vi "cm2nm_read_session_data_file_backup.vi"(2 "TopLevelDataFilePath":path, 3 "Session_data_base":path) -> (0 "error out":errorcluster, 1 "Sample Set":T6)   [LabVIEW 2010]
uses:
  cm2nm_sample_set.ctl
  cm2nm_coordinate_information_v2.ctl
  Instrument_type_enum_v2.ctl
  cm2nm_sample_set_old_1.ctl
  Instrument_type_enum.ctl
  <vilib>/Utility/xml.llb/Read From XML File(string).vi
panel:
  out "Sample Set 4":T1
  out "Sample Set 3":T4
  in  "Sample Set 2":T5
  out "String":string
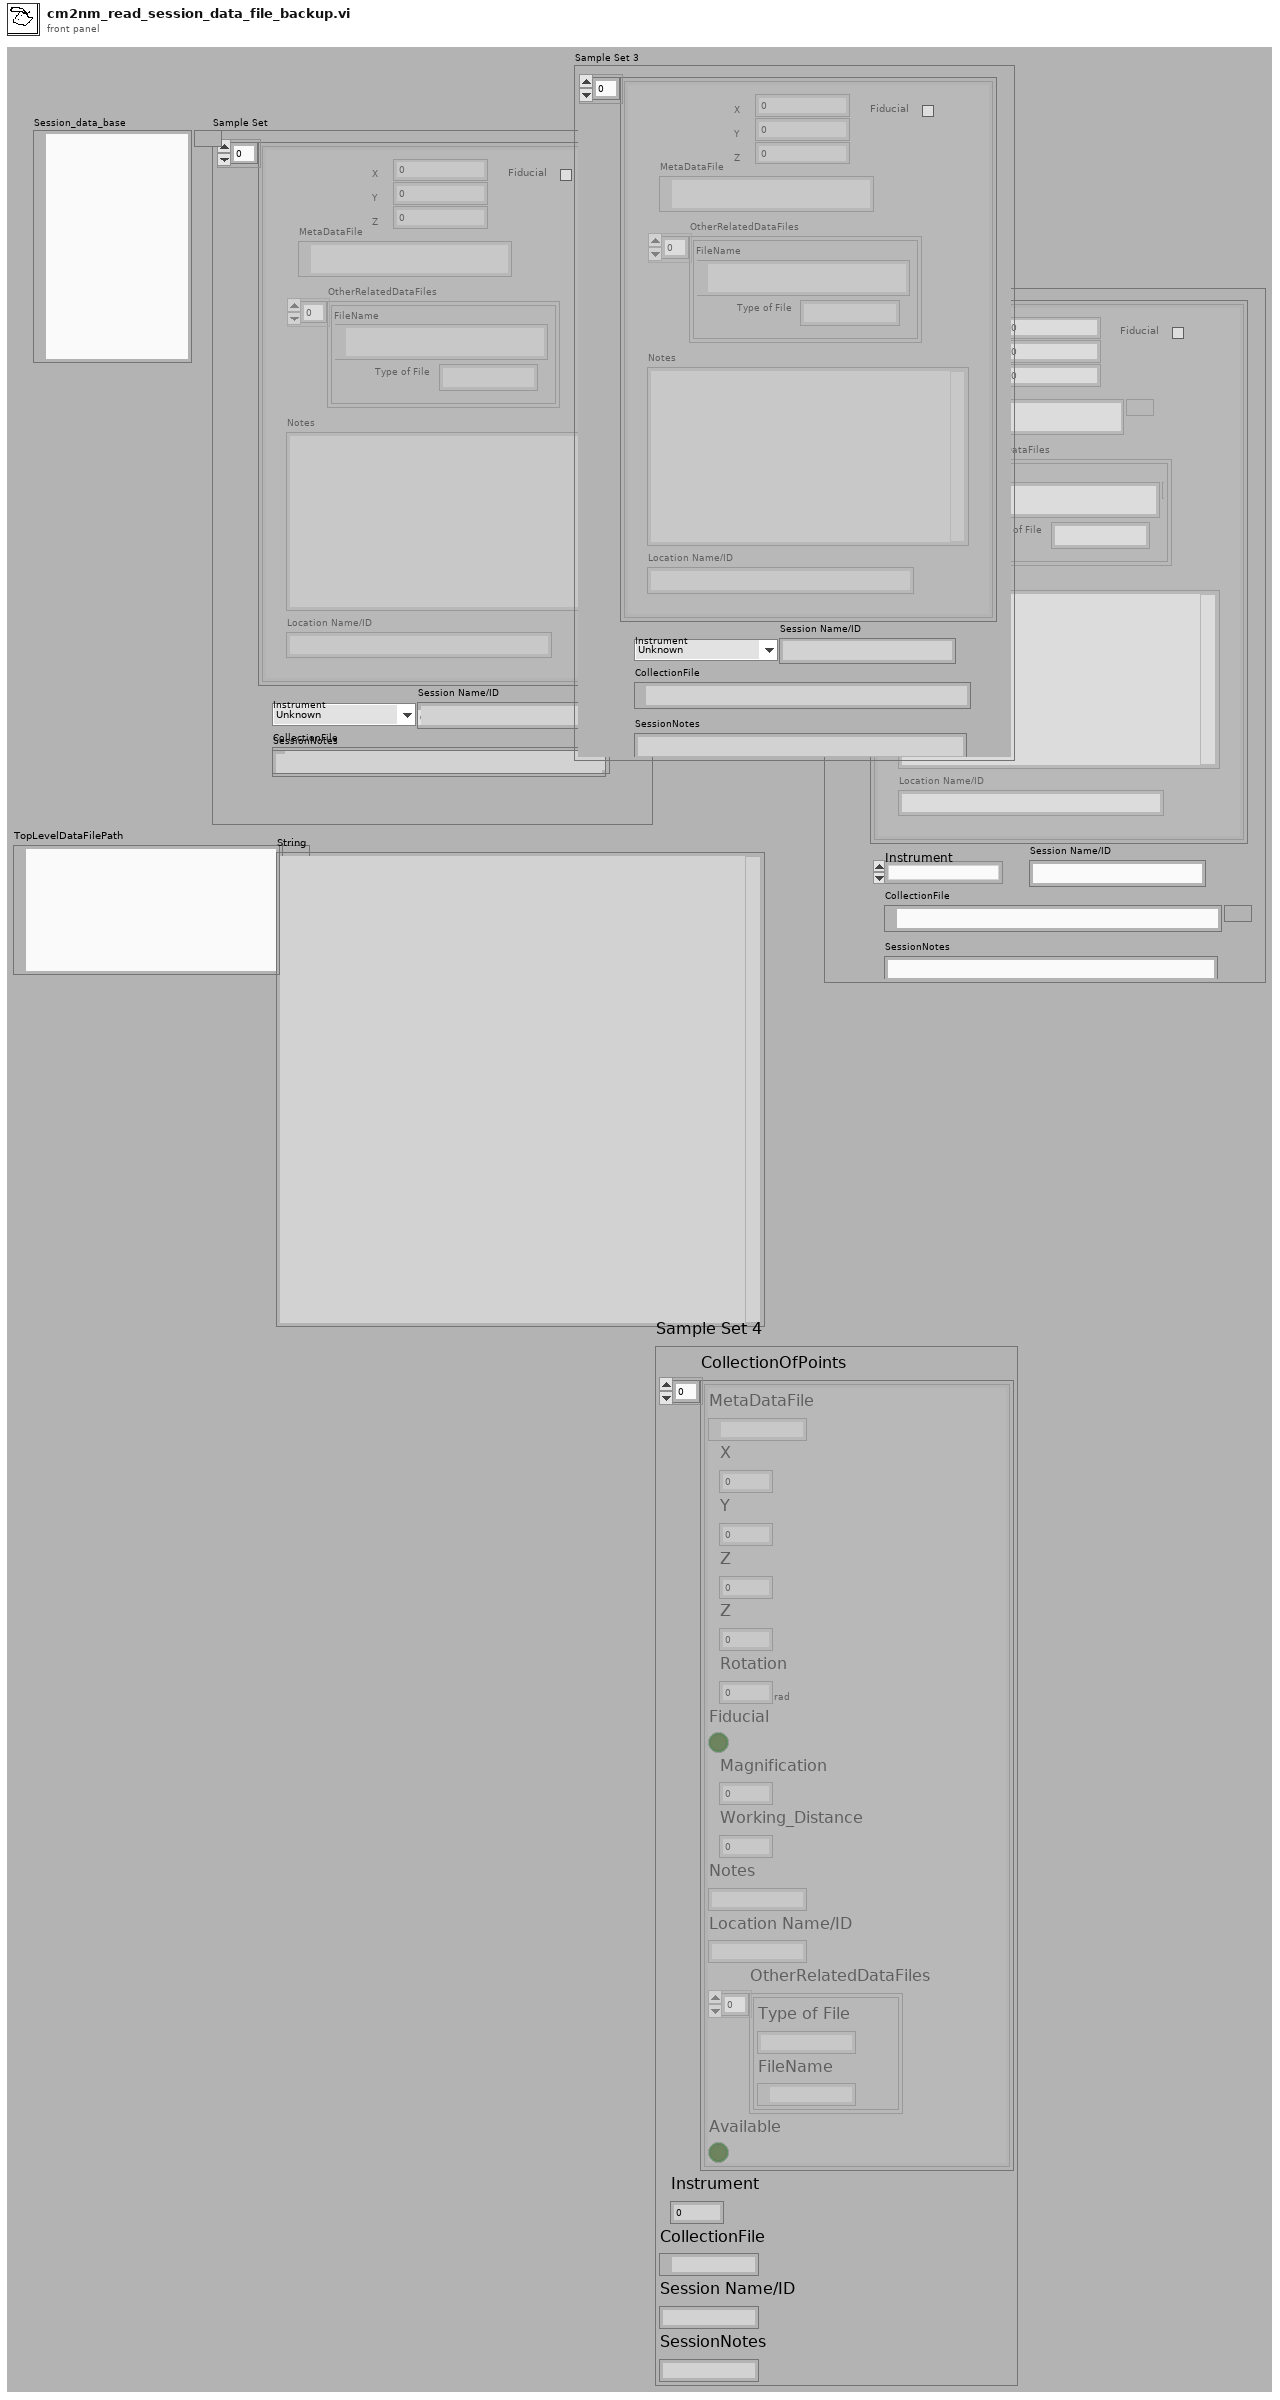
[diagram p1: front panel]
types:
  T1 = cluster{"CollectionOfPoints":cluster{"MetaDataFile":path, "X":dbl, "Y":dbl, "Z":dbl, "Z":dbl, "Rotation":dbl[unit], "Fiducial":bool, "Magnification":dbl, "Working_Distance":dbl, "Notes":string, "Location Name/ID":string, "OtherRelatedDataFiles":cluster{"Type of File":string, "FileName":path}[], "Available":bool}[], "Instrument":u16, "CollectionFile":path, "Session Name/ID":string, "SessionNotes":string}
  T2 = typedef "cm2nm_coordinate_information_v2.ctl" = cluster{"MetaDataFile":path, "X":dbl, "Y":dbl, "Z":dbl, "Group":i32, "Rotation":dbl[unit], "Fiducial":bool, "Magnification":dbl, "Working_Distance":dbl, "Notes":string, "Location Name/ID":string, "OtherRelatedDataFiles":cluster{"Type of File":string, "FileName":path}[], "Available":bool}
  T3 = typedef "Instrument_type_enum.ctl" = enum16{"Unknown", "Phillips FEI SEM IRC", "JEOL 7000F EML_MFC", "MXRD MFC", "JEOL_EPMA"}
  T4 = cluster{"CollectionOfPoints":T2[], "Instrument":T3, "CollectionFile":path, "Session Name/ID":string, "SessionNotes":string}
  T5 = typedef "cm2nm_sample_set_old_1.ctl" = cluster{"CollectionOfPoints":T2[], "Instrument":enum16{""}, "CollectionFile":path, "Session Name/ID":string, "SessionNotes":string}
  T6 = typedef "cm2nm_sample_set.ctl" = cluster{"CollectionOfPoints":T2[], "Instrument":T7, "CollectionFile":path, "Session Name/ID":string, "SessionNotes":string}
  T7 = typedef "Instrument_type_enum_v2.ctl" = enum16{"Unknown", "Philips FEI SEM IRC", "JEOL 7000F EML_MFC", "MXRD MFC", "JEOL_EPMA"}
  T8 = cluster{"CollectionOfPoints":cluster{"MetaDataFile":path, "X":dbl, "Y":dbl, "Group":i32, "Z":dbl, "Rotation":dbl[unit], "Fiducial":bool, "Magnification":dbl, "Working_Distance":dbl, "Notes":string, "Location Name/ID":string, "OtherRelatedDataFiles":cluster{"Type of File":string, "FileName":path}[], "Available":bool}[], "Instrument":T7, "CollectionFile":path, "Session Name/ID":string, "SessionNotes":string}
  T9 = cluster{"CollectionOfPoints":cluster{"MetaDataFile":path, "X":dbl, "Y":dbl, "Z":dbl, "Group":i32, "Rotation":dbl[unit], "Fiducial":bool, "Magnification":dbl, "Working_Distance":dbl, "Notes":string, "Location Name/ID":string, "OtherRelatedDataFiles":cluster{"Type of File":string, "FileName":path}[], "Available":bool}[], "Instrument":T3, "CollectionFile":path, "Session Name/ID":string, "SessionNotes":string}
  T10 = cluster{"MetaDataFile":path, "X":dbl, "Y":dbl, "Z":dbl, "Group":i32, "Rotation":dbl[unit], "Fiducial":bool, "Magnification":dbl, "Working_Distance":dbl, "Notes":string, "Location Name/ID":string, "OtherRelatedDataFiles":cluster{"Type of File":string, "FileName":path}[], "Available":bool}[]
  T11 = cluster{"MetaDataFile":path, "X":dbl, "Y":dbl, "Group":i32, "Z":dbl, "Rotation":dbl[unit], "Fiducial":bool, "Magnification":dbl, "Working_Distance":dbl, "Notes":string, "Location Name/ID":string, "OtherRelatedDataFiles":cluster{"Type of File":string, "FileName":path}[], "Available":bool}[]
  T12 = cluster{"CollectionOfPoints":cluster{"MetaDataFile":path, "X":dbl, "Y":dbl, "Group":i32, "Z":dbl, "Rotation":dbl[unit], "Fiducial":bool, "Magnification":dbl, "Working_Distance":dbl, "Notes":string, "Location Name/ID":string, "OtherRelatedDataFiles":cluster{"Type of File":string, "FileName":path}[], "Available":bool}[], "Instrument":u16, "CollectionFile":path, "Session Name/ID":string, "SessionNotes":string}
  T13 = cluster{"MetaDataFile":path, "X":dbl, "Y":dbl, "Z":dbl, "Z":dbl, "Rotation":dbl[unit], "Fiducial":bool, "Magnification":dbl, "Working_Distance":dbl, "Notes":string, "Location Name/ID":string, "OtherRelatedDataFiles":cluster{"Type of File":string, "FileName":path}[], "Available":bool}[]
  T14 = cluster{"MetaDataFile":path, "X":dbl, "Y":dbl, "Z":dbl, "Z":dbl, "Rotation":dbl[unit], "Fiducial":bool, "Magnification":dbl, "Working_Distance":dbl, "Notes":string, "Location Name/ID":string, "OtherRelatedDataFiles":cluster{"Type of File":string, "FileName":path}[], "Available":bool}
  T15 = cluster{"CollectionOfPoints":cluster{"MetaDataFile":path, "X":dbl, "Y":dbl, "Z":dbl, "Z":dbl, "Rotation":dbl[unit], "Fiducial":bool, "Magnification":dbl, "Working_Distance":dbl, "Notes":string, "Location Name/ID":string, "OtherRelatedDataFiles":cluster{"Type of File":string, "FileName":path}[], "Available":bool}[], "Instrument":T7, "CollectionFile":path, "Session Name/ID":string, "SessionNotes":string}
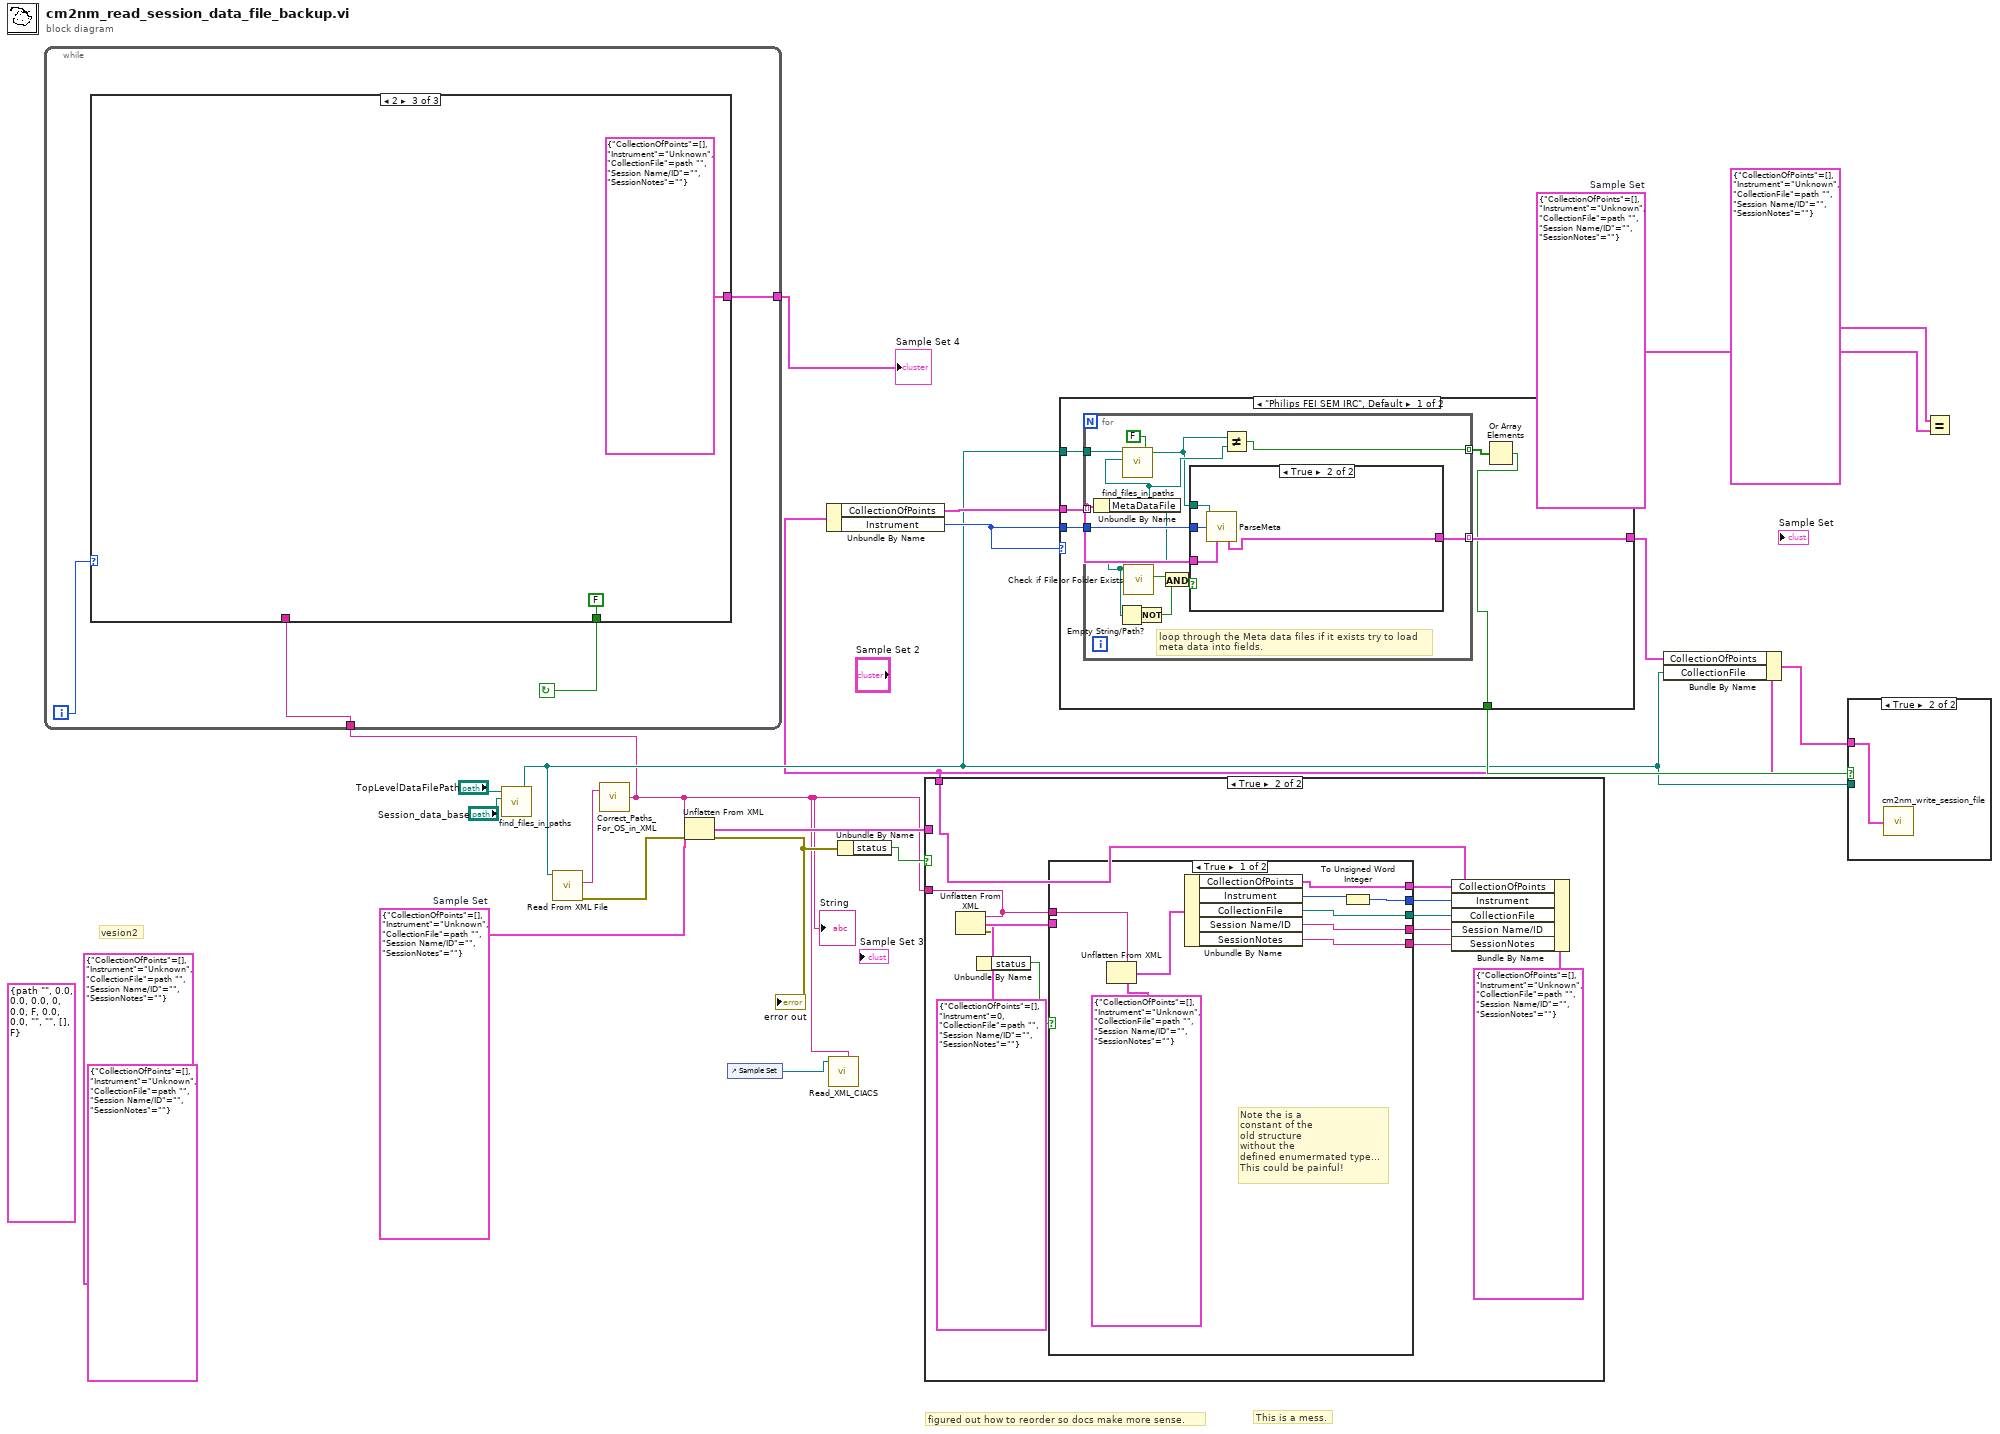
[diagram p0: block diagram]
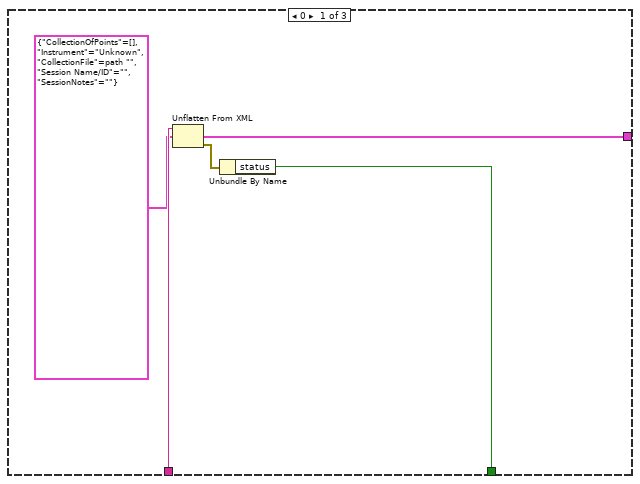
[diagram p2: hidden frame]
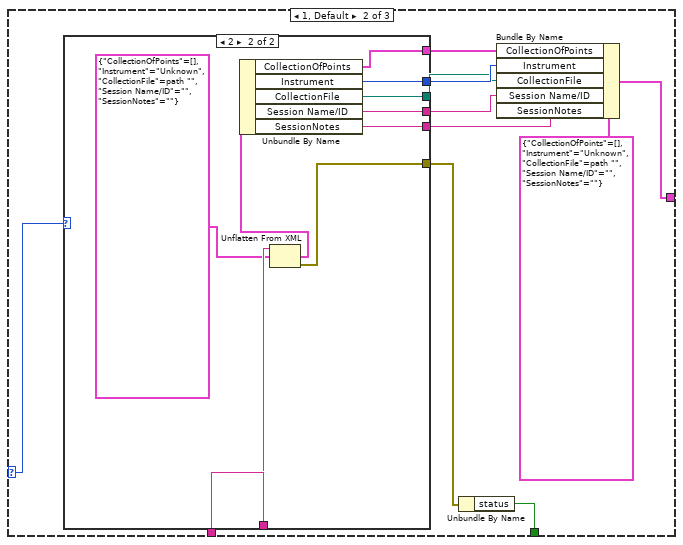
[diagram p3: hidden frame]
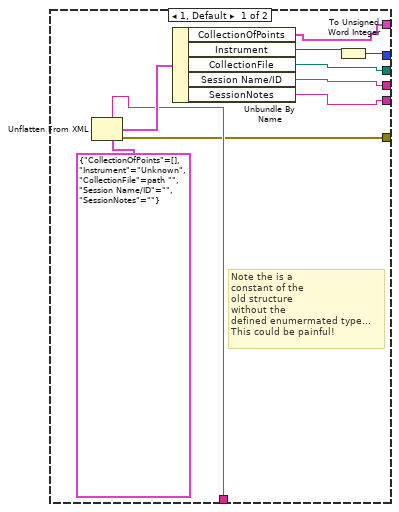
[diagram p4: hidden frame]
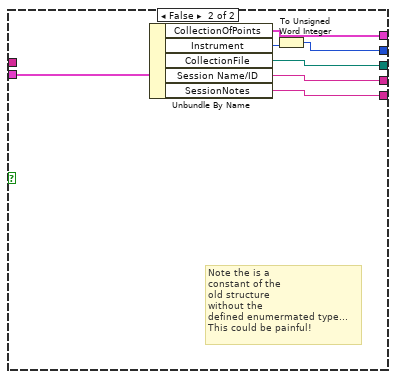
[diagram p6: hidden frame]
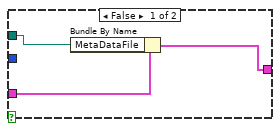
[diagram p8: hidden frame]
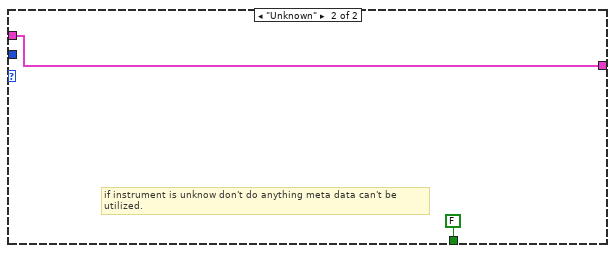
[diagram p9: hidden frame]
diagram:
  (unwired) T2 {"MetaDataFile"=path "", "X"=0.0, "Y"=0.0, "Z"=0.0, "Group"=0, "Rotation"=0.0, "Fiducial"=FALSE, "Magnification"=0.0, "Working_Distance"=0.0, "Notes"="", "Location Name/ID"="", "OtherRelatedDataFiles"=[], "Available"=FALSE} ("Cluster")
  (unwired) T6 {"CollectionOfPoints"=[], "Instrument"=enum."Unknown", "CollectionFile"=path "", "Session Name/ID"="", "SessionNotes"=""} ("value")
  (unwired) T6 {"CollectionOfPoints"=[], "Instrument"=enum."Unknown", "CollectionFile"=path "", "Session Name/ID"="", "SessionNotes"=""} ("Sample Set")
  w10 = T6 {"CollectionOfPoints"=[], "Instrument"=enum."Unknown", "CollectionFile"=path "", "Session Name/ID"="", "SessionNotes"=""}  # Sample Set
  w4 = T8 {"CollectionOfPoints"=[], "Instrument"=enum."Unknown", "CollectionFile"=path "", "Session Name/ID"="", "SessionNotes"=""}  # Sample Set
  # "This is a mess."
  # "figured out how to reorder so docs make more sense."
  # "vesion2"
  n1 = call "find_files_in_paths.vi"("TopLevelDataFilePath"="TopLevelDataFilePath", "subbordinateFilePath"="Session_data_base") -> ("Path"=w12:path)  [unwired: 4 in, 1 out]
  n2 = call-poly <vilib>:"Read From XML File.vi"("XML File Path"=w12) -> ("error out"=w20:errorcluster, "XML Elements"=w15:string)  [unwired: 1 in, 8 out]
  n3 = call "Correct_Paths_For_OS_in_XML.vi"("XML Elements"=w15) -> ("String"=w2:string)  [unwired: 1 in]
  "String" <- w2
  n4 = while {
    tunnel: w2 -> [w23]
    tunnel: [w22] -> w3
    i -> [w24]
    stop <- w21 continue-if-true
    n5 = case shown="2" w24 {
      selector: w24 -> [_ w39 _]
      tunnel: w23 -> [w29 w38 _]
      tunnel: [w27 w32 T6 {"CollectionOfPoints"=[], "Instrument"=enum."Unknown", "CollectionFile"=path "", "Session Name/ID"="", "SessionNotes"=""} ("Sample Set")] -> w22
      tunnel: [w25 w31 FALSE ("status")] -> w21
      frame 0 {
        n6 = Unflatten From XML(xml string=w29, type=T6 {"CollectionOfPoints"=[], "Instrument"=enum."Unknown", "CollectionFile"=path "", "Session Name/ID"="", "SessionNotes"=""} ("Sample Set")) -> (value=w27:T6, error out=w26:errorcluster)  [unwired: 1 in]
        n7 = Unbundle By Name(w26) -> ("status"=w25:bool)
      }
      frame 1, Default {
        n8 = case shown="2" w39 {
          tunnel: w38 -> [w47 w59]
          tunnel: [w46 w56] -> w37
          tunnel: [w45 w55] -> w36
          tunnel: [w44 w54] -> w35
          tunnel: [w43 w53] -> w34
          tunnel: [w42 w52] -> w33
          tunnel: [w41 w51] -> w30
          frame 1, Default {
            # "Note the is a \nconstant of the\nold structure\nwithout the\ndefined enumermated type...\nThis could be painful!"
            n9 = Unflatten From XML(xml string=w47, type=T9 {"CollectionOfPoints"=[], "Instrument"=enum."Unknown", "CollectionFile"=path "", "Session Name/ID"="", "SessionNotes"=""} ("Sample Set 3")) -> (value=w50:T9, error out=w41:errorcluster)  [unwired: 1 in]
            n10 = Unbundle By Name(w50) -> ("CollectionOfPoints"=w46:T10, "Instrument"=w48:T3, "CollectionFile"=w44:path, "Session Name/ID"=w43:string, "SessionNotes"=w42:string)
            n11 = To Unsigned Word Integer(number=w48) -> (unsigned 16bit integer=w45:u16)
          }
          frame 2 {
            n12 = Unflatten From XML(xml string=w59, type=T8 {"CollectionOfPoints"=[], "Instrument"=enum."Unknown", "CollectionFile"=path "", "Session Name/ID"="", "SessionNotes"=""} ("Sample Set")) -> (value=w57:T8, error out=w51:errorcluster)  [unwired: 1 in]
            n13 = Unbundle By Name(w57) -> ("CollectionOfPoints"=w56:T11, "Instrument"=w55:T7, "CollectionFile"=w54:path, "Session Name/ID"=w53:string, "SessionNotes"=w52:string)
          }
        }
        n14 = Unbundle By Name(w30) -> ("status"=w31:bool)
        n15 = Bundle By Name(cluster=T6 {"CollectionOfPoints"=[], "Instrument"=enum."Unknown", "CollectionFile"=path "", "Session Name/ID"="", "SessionNotes"=""} ("Sample Set"), "CollectionOfPoints"=w37, "Instrument"=w36, "CollectionFile"=w35, "Session Name/ID"=w34, "SessionNotes"=w33) -> (w32:T6)
      }
      frame 2 {
      }
    }
  }
  "Sample Set 4" <- w3
  n16 = Unflatten From XML(xml string=w2, type=w4, error in (no error)=w20) -> (value=w7:T8, error out=w8:errorcluster)
  "error out" <- w8
  n17 = control-ref of="Sample Set"() -> (w1:refnum<vi>)
  n18 = call "Read_XML_CIACS.vi"("XML_Cluster_String"=w2, "Sample Set"=w1) -> ()  [unwired: 7 out]
  n19 = Unbundle By Name(w8) -> ("status"=w6:bool)
  n20 = case shown="True" w6 {
    tunnel: w7 -> [w62 _]
    tunnel: [w62 w67] -> w5
    tunnel: w2 -> [_ w63]
    frame False {
    }
    frame True {
      n21 = Unflatten From XML(xml string=w63, type=T12 {"CollectionOfPoints"=[], "Instrument"=0, "CollectionFile"=path "", "Session Name/ID"="", "SessionNotes"=""} ("Sample Set")) -> (value=w74:T12, error out=w65:errorcluster)  [unwired: 1 in]
      n22 = Unbundle By Name(w65) -> ("status"=w64:bool)
      n23 = case shown="True" w64 {
        tunnel: w74 -> [_ w90]
        tunnel: [w83 w89] -> w72
        tunnel: [w82 w88] -> w71
        tunnel: [w81 w87] -> w70
        tunnel: [w80 w86] -> w69
        tunnel: [w78 w84] -> w68
        tunnel: w63 -> [w77 _]
        frame True {
          # "Note the is a \nconstant of the\nold structure\nwithout the\ndefined enumermated type...\nThis could be painful!"
          n24 = Unflatten From XML(xml string=w77, type=T9 {"CollectionOfPoints"=[], "Instrument"=enum."Unknown", "CollectionFile"=path "", "Session Name/ID"="", "SessionNotes"=""} ("Sample Set 3")) -> (value=w75:T9)  [unwired: 1 in, 1 out]
          n25 = Unbundle By Name(w75) -> ("CollectionOfPoints"=w83:T10, "Instrument"=w79:T3, "CollectionFile"=w82:path, "Session Name/ID"=w81:string, "SessionNotes"=w80:string)
          n26 = To Unsigned Word Integer(number=w79) -> (unsigned 16bit integer=w78:u16)
        }
        frame False {
          # "Note the is a \nconstant of the\nold structure\nwithout the\ndefined enumermated type...\nThis could be painful!"
          n27 = Unbundle By Name(w90) -> ("CollectionOfPoints"=w89:T11, "Instrument"=w85:u16, "CollectionFile"=w88:path, "Session Name/ID"=w87:string, "SessionNotes"=w86:string)
          n28 = To Unsigned Word Integer(number=w85) -> (unsigned 16bit integer=w84:u16)
        }
      }
      n29 = Bundle By Name(cluster=T6 {"CollectionOfPoints"=[], "Instrument"=enum."Unknown", "CollectionFile"=path "", "Session Name/ID"="", "SessionNotes"=""} ("Sample Set"), "CollectionOfPoints"=w72, "Instrument"=w68, "CollectionFile"=w71, "Session Name/ID"=w70, "SessionNotes"=w69) -> (w67:T6)
    }
  }
  n30 = Unbundle By Name(w5) -> ("CollectionOfPoints"=w19:T13, "Instrument"=w17:T7)
  n31 = case shown="\"Philips FEI SEM IRC\", Default" w17 {
    tunnel: w19 -> [w96 w117]
    tunnel: w17 -> [w95 _]
    tunnel: [w94 w117] -> w18
    tunnel: w12 -> [w92 _]
    tunnel: [w91 FALSE] -> w16
    frame "Philips FEI SEM IRC", Default {
      n32 = for {
        tunnel: w96 -> [w107] mode=indexing
        tunnel: w95 -> [w108]
        tunnel: [w106] -> w94 mode=indexing
        tunnel: w92 -> [w101]
        tunnel: [w97] -> w93 mode=indexing
        # "loop through the Meta data files if it exists try to load\nmeta data into fields."
        n33 = Unbundle By Name(w107) -> ("MetaDataFile"=w99:path)
        n34 = Empty String/Path?(string/path=w99) -> (empty?=w105:bool)
        n35 = call "find_files_in_paths.vi"("TopLevelDataFilePath"=w101, "subbordinateFilePath"=w99, "PromptFormissingFile"=FALSE) -> ("Path"=w98:path)  [unwired: 3 in, 1 out]
        n36 = call <vilib>:"Check if File or Folder Exists.vi"("path"=w99) -> ("file or folder exists?"=w102:bool)  [unwired: 1 in, 9 out]
        n37 = Not(x=w105) -> (.not. x?=w103:bool)
        n38 = And(x=w102, y=w103) -> (x .and. y?=w104:bool)
        n39 = case shown="True" w104 {
          tunnel: w108 -> [_ w115]
          tunnel: w98 -> [w110 w114]
          tunnel: w107 -> [w111 w113]
          tunnel: [w109 w112] -> w106
          frame False {
            n40 = Bundle By Name(cluster=w111, "MetaDataFile"=w110) -> (w109:T14)
          }
          frame True {
            n41 = call "ParseMeta.vi"("Path"=w114, "Instrument"=w115, "Spot_info_in"=w113) -> ("Spot_info_out"=w112:T2)  [unwired: 12 out]
          }
        }
        n42 = Not Equal?(x=w98, y=w99) -> (x != y?=w97:bool)
      }
      n43 = Or Array Elements(Boolean array=w93) -> (logical OR=w91:bool)
    }
    frame "Unknown" {
      # "if instrument is unknow don't do anything meta data can't be\nutilized."
    }
  }
  n44 = Bundle By Name(cluster=w5, "CollectionOfPoints"=w18, "CollectionFile"=w12) -> (w9:T15)
  n45 = case shown="True" w16 {
    tunnel: w12 -> [_ _]
    tunnel: w9 -> [_ w118]
    frame False {
    }
    frame True {
      n46 = call "cm2nm_write_session_file.vi"("Session Information"=w118) -> ()  [unwired: 1 out]
    }
  }
  n47 = Equal?(x=T6 {"CollectionOfPoints"=[], "Instrument"=enum."Unknown", "CollectionFile"=path "", "Session Name/ID"="", "SessionNotes"=""} ("output cluster"), y=w10) -> ()  [unwired: 1 out]
